vi "Create Helper Loop Events.vi"(11 "Acquisition UI in":refnum<class "Acquisition UI.lvclass">) -> (3 "Acquisition UI out":refnum<class "Acquisition UI.lvclass">)   [LabVIEW 2018, in "Acquisition UI.lvlib" / "Acquisition UI.lvclass"]
uses:
  Acquisition UI.lvclass
  Acquisition UI.lvclass/Acquisition UI.ctl
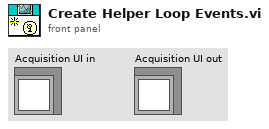
[diagram p1: front panel]
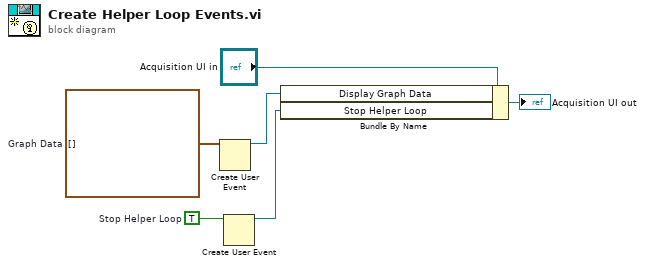
[diagram p0: block diagram]
diagram:
  w3 = TRUE  # Stop Helper Loop
  w2 = waveform(dbl)[] []  # Graph Data
  n1 = Create User Event(user event datatype=w2) -> (user event=w5:refnum<user-event>)  [unwired: 1 in, 1 out]
  n2 = Create User Event(user event datatype=w3) -> (user event=w6:refnum<user-event>)  [unwired: 1 in, 1 out]
  n3 = Bundle By Name(cluster="Acquisition UI in", "Display Graph Data"=w5, "Stop Helper Loop"=w6) -> (→"Acquisition UI out":refnum<class "Acquisition UI.lvclass">)
